vi "Thermocouple Junction Temperature Data.vi"(8 "error in (no error)":errorcluster, 11 "VISA resource name":refnum<visa-resource-name>) -> (0 "error out":errorcluster, 2 "Room-Temperature Sensor Data":dbl format="%.1f", 3 "VISA resource name out":refnum<visa-resource-name>)   [LabVIEW 2019, in "Lake Shore 335.lvlib"]
doc: "This VI returns the temperature reading in Kelvin measured by the built-in room-temperature compensation sensor."
uses:
  Lake Shore 335.lvlib
  Instance           1 46Saved   Thermocouple Junction Temperature Data .vi
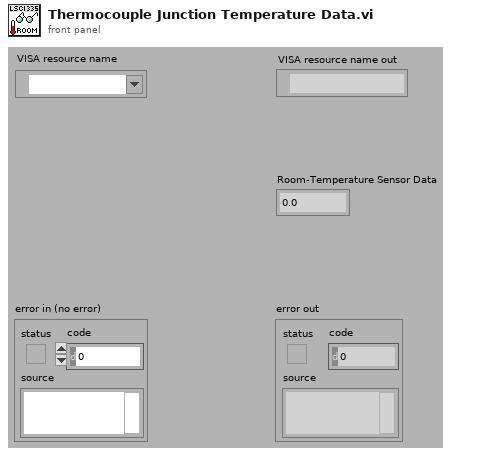
[diagram p1: front panel]
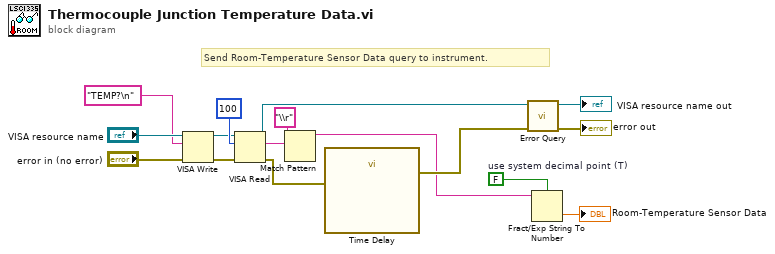
[diagram p0: block diagram]
diagram:
  w5 = FALSE  # use system decimal point (T)
  # "Send Room-Temperature Sensor Data query to instrument."
  n1 = VISA Write(VISA resource name="VISA resource name", write buffer="TEMP?\n", error in (no error)="error in (no error)") -> (VISA resource name out=w12:refnum<visa-resource-name>, error out=w11:errorcluster)  [unwired: 1 out]
  n2 = VISA Read(VISA resource name=w12, byte count=100, error in (no error)=w11) -> (VISA resource name out=w8:refnum<visa-resource-name>, read buffer=w14:string, error out=w10:errorcluster)  [unwired: 1 out]
  n3 = Match Pattern(string=w14, regular expression="\\r") -> (before substring=w4:string)  [unwired: 1 in, 3 out]
  n4 = call "Time Delay"("error in (no error)"=w10) -> ("error out"=w9:errorcluster)  [unwired: 10 in]
  n5 = call "Error Query.vi"("error in (no error)"=w9, "VISA resource name"=w8) -> ("error out"=→"error out":errorcluster, "VISA resource name out"=→"VISA resource name out":refnum<visa-resource-name>)  [unwired: 7 in, 1 out]
  n6 = Fract/Exp String To Number(use system decimal point (T)=w5, string=w4) -> (number=→"Room-Temperature Sensor Data":dbl)  [unwired: 2 in, 1 out]
